vi "LinxUartClose.vi"(8 "Error In":errorcluster, 10 "Uart Channel":u8, 11 "LINX Resource":T1) -> (0 "Error Out":errorcluster, 3 "LINX Resource":T1)   [LabVIEW 2014, in "LMH-LINX.lvlib" / "Local IO.lvlib"]
uses:
  <vilib>/MakerHub/LINX/Private/Local IO/Local IO.lvlib
  <vilib>/MakerHub/LINX/Private/Type Defs/LINX Ref.ctl
  <vilib>/MakerHub/LINX/Private/Type Defs/Platform.ctl
  <vilib>/MakerHub/LINX/Private/Type Defs/Interface.ctl
  <vilib>/MakerHub/LINX/Private/Device/Type Defs/LINX Device Config.ctl
  <vilib>/MakerHub/LINX/Private/Device/Type Defs/TCP Config.ctl
  <vilib>/MakerHub/LINX/Private/Device/Type Defs/Channels.ctl
  <vilib>/MakerHub/LINX/Private/Type Defs/Error Type.ctl
  <vilib>/MakerHub/LINX/LMH-LINX.lvlib
  <vilib>/MakerHub/LINX/Private/Type Defs/Channel FGV States.ctl
  liblinxdevice.dll
  <vilib>/MakerHub/LINX/Private/Device/Device.lvlib
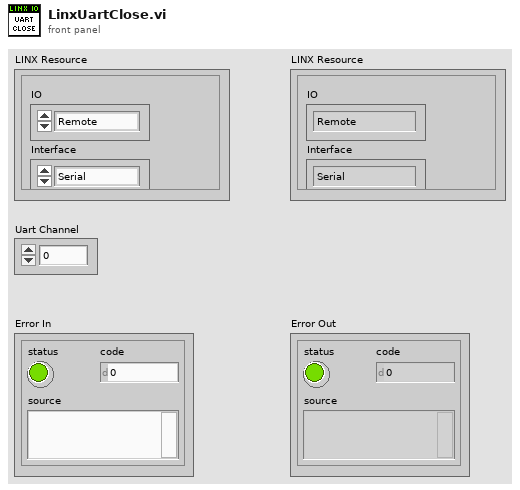
[diagram p1: front panel]
types:
  T1 = typedef "LMH-LINX.lvlib/LINX Ref.ctl" = cluster{"IO":T2, "Interface":T3, "LINX Device Config":T4}
  T2 = typedef "LMH-LINX.lvlib/Platform.ctl" = enum16{"Remote", "Local"}
  T3 = typedef "LMH-LINX.lvlib/Interface.ctl" = enum16{"Serial", "TCP"}
  T4 = typedef "LMH-LINX.lvlib/Device.lvlib/LINX Device Config.ctl" = cluster{"Interface":T3, "COM Port":refnum<visa-resource-name>, "TCP Configuration":T5, "Device Family":u8, "Device ID":u8, "Device Name":string, "TCP Ref":refnum<k5>, "Channels":T6}
  T5 = typedef "LMH-LINX.lvlib/Device.lvlib/TCP Config.ctl" = cluster{"IP Address":string, "Port":u16}
  T6 = typedef "LMH-LINX.lvlib/Channels.ctl" = cluster{"DI":u8[], "DO":u8[], "AI":u8[], "AO":u8[], "PWM":u8[], "QE":u8[], "UART":u8[], "I2C 2":u8[], "SPI":u8[], "CAN":u8[], "Servo":u8[], "AI Ref (V)":dbl, "AI Resolution (Bits)":u8, "AO Ref (V)":dbl, "AO Resolution (Bits)":u8}
  T7 = typedef "LMH-LINX.lvlib/Error Type.ctl" = enum16{"Unknown", "Timeout", "Corrupt Return Packet", "Unable To Connect", "Command Not Supported", "Channel DNE", "Invalid COM Config", "Firmware Version Mismatch", "myRIO Support", "CMD Specific Error", "Local IO Not Supported"}
  T8 = typedef "LMH-LINX.lvlib/Channel FGV States.ctl" = enum16{"Initialize", "Get", "Set"}
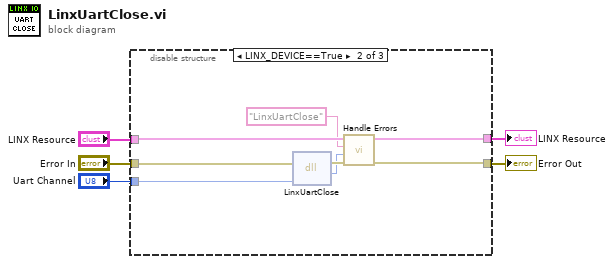
[diagram p0: block diagram]
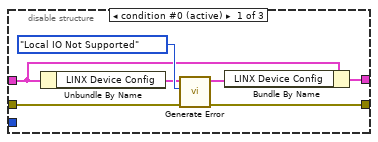
[diagram p2: hidden frame]
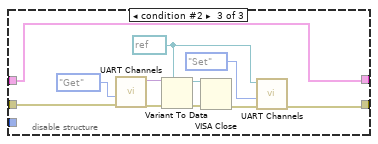
[diagram p3: hidden frame]
diagram:
  n1 = disable-structure shown="LINX_DEVICE==True" {
    disable-tunnel: [w6 w17 w22] -> w4
    disable-tunnel: "LINX Resource" -> [w8 w18 w22]
    disable-tunnel: "Error In" -> [w11 w20 w21]
    disable-tunnel: [w10 w15 w23] -> w5
    disable-tunnel: "Uart Channel" -> [_ w19 _]
    frame condition #0 (active) {
      n2 = Unbundle By Name(w8) -> ("LINX Device Config"=w9:T4)
      n3 = call <vilib>:"Generate Error.vi"("Error In"=w11, "Error Type"=Error_Type."Local IO Not Supported", "LINX Device Config"=w9) -> ("Error Out"=w10:errorcluster, "Dup LINX Device Config"=w7:T4)  [unwired: 7 in]
      n4 = Bundle By Name(cluster=w8, "LINX Device Config"=w7) -> (w6:T1)
    }
    frame condition #1 {
      n5 = dll-call lib="liblinxdevice.*" fn="LinxUartClose"(error in=w20, "channel"=w19) -> (error out=w16:errorcluster, "status"=w13:i32)  [unwired: 3 in, 1 out]
      n6 = call <vilib>:"Handle Errors.vi"("Error In"=w16, "LinxStatus"=w13, "Function Name"="LinxUartClose", "LINX Resource"=w18) -> ("Error Out"=w15:errorcluster, "LINX Resource"=w17:T1)  [unwired: 6 in]
    }
    frame condition #2 {
      w31 = refnum<visa-resource-name> refnum ("VISA resource name")
      n7 = call <vilib>:"UART Channels.vi"("Error In"=w21, "Channel State"=Channel_FGV_States."Get") -> ("Error Out"=w27:errorcluster, "UART Channel"=w28:variant)  [unwired: 8 in]
      n8 = Variant To Data(error in=w27, type=w31, Variant=w28) -> (data=w29:refnum<visa-resource-name>, error out=w26:errorcluster)
      n9 = VISA Close(VISA resource name=w29, error in (no error)=w26) -> (error out=w30:errorcluster)
      n10 = call <vilib>:"UART Channels.vi"("Error In"=w30, "Channel State"=Channel_FGV_States."Set", "UART Channel"=w31) -> ("Error Out"=w23:errorcluster)  [unwired: 7 in, 1 out]
    }
  }
  "LINX Resource" <- w4
  "Error Out" <- w5
